vi "NRCToString.vi"(3 "SIDRQ":u8) -> (1 "NRC Message":string)   [LabVIEW 2011, in "Konvolucio MUDS150628.lvlib"]
uses:
  <instrlib>/Konvolucio MUDS150628/Konvolucio MUDS150628.lvlib
panel:
  out "NRC Num":T1(ring)=enum."noResponseFromSubnetComponent"
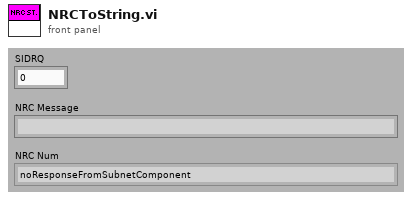
[diagram p1: front panel]
types:
  T1 = enum16{"generalReject", "serviceNotSupported", "subFunctionNotSupported", "incorrectMessageLengthOrInvalidFormat", "responseTooLong", "busyRepeatRequest", "conditionsNotCorrect", "requestSequenceError", "noResponseFromSubnetComponent", "failurePreventsExecutionOfRequestedAction", "requestOutOfRange", "securityAccessDenied", "invalidKey", "exceedNumberOfAttempts", "requiredTimeDelayNotExpired", "uploadDownloadNotAccepted", "transferDataSuspended", "generalProgrammingFailure", "wrongBlockSequenceCounter", "requestCorrectlyReceived", "subFunctionNotSupportedInActiveSession", "serviceNotSupportedInActiveSession", "rpmTooHigh", "rpmTooLow", "engineIsRunning", "engineIsNotRunning", "engineRunTimeTooLow", "temperatureTooHigh", "temperatureTooLow", "vehicleSpeedTooHigh", "vehicleSpeedTooLow", "throttle/PedalTooHigh", "throttle/PedalTooLow", "transmissionRangeNotInNeutral", "transmissionRangeNotInGear", "brakeSwitch(es)NotClosed", "shifterLeverNotInPark", "torqueConverterClutchLocked", "voltageTooHigh", "voltageTooLow", "undefined"}
  T2 = enum16{"generalReject", "serviceNotSupported", "subFunctionNotSupported", "incorrectMessageLengthOrInvalidFormat", "responseTooLong", "busyRepeatRequest", "conditionsNotCorrect", "requestSequenceError", "noResponseFromSubnetComponent", "failurePreventsExecutionOfRequestedAction", "requestOutOfRange", "securityAccessDenied", "invalidKey", "exceedNumberOfAttempts", "requiredTimeDelayNotExpired", "uploadDownloadNotAccepted", "transferDataSuspended", "generalProgrammingFailure", "wrongBlockSequenceCounter", "requestCorrectlyReceived", "subFunctionNotSupportedInActiveSession", "serviceNotSupportedInActiveSession", "rpmTooHigh", "rpmTooLow", "engineIsRunning", "engineIsNotRunning", "engineRunTimeTooLow", "temperatureTooHigh", "temperatureTooLow", "vehicleSpeedTooHigh", "vehicleSpeedTooLow", "throttle/PedalTooHigh", "throttle/PedalTooLow", "transmissionRangeNotInNeutral", "transmissionRangeNotInGear", "brakeSwitch(es)NotClosed", "shifterLeverNotInPark", "torqueConverterClutchLocked", "voltageTooHigh", "voltageTooLow"}
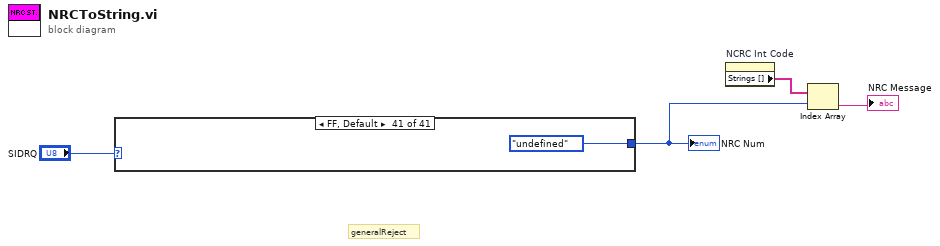
[diagram p0: block diagram]
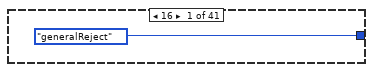
[diagram p2: hidden frame]
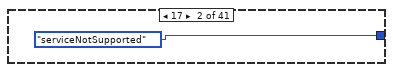
[diagram p3: hidden frame]
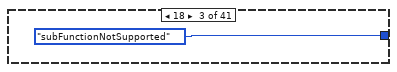
[diagram p4: hidden frame]
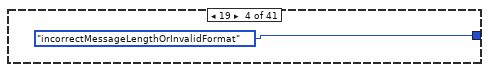
[diagram p5: hidden frame]
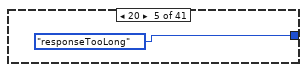
[diagram p6: hidden frame]
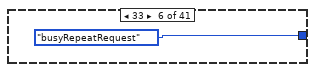
[diagram p7: hidden frame]
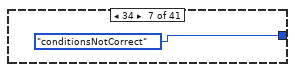
[diagram p8: hidden frame]
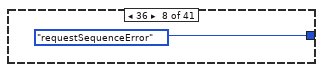
[diagram p9: hidden frame]
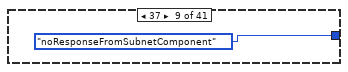
[diagram p10: hidden frame]
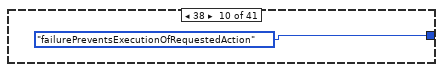
[diagram p11: hidden frame]
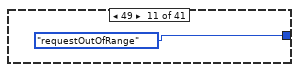
[diagram p12: hidden frame]
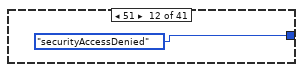
[diagram p13: hidden frame]
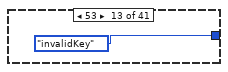
[diagram p14: hidden frame]
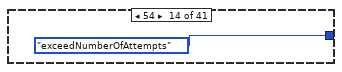
[diagram p15: hidden frame]
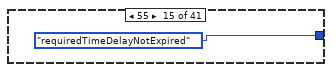
[diagram p16: hidden frame]
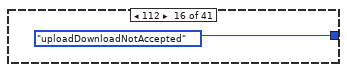
[diagram p17: hidden frame]
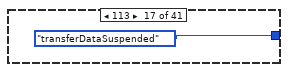
[diagram p18: hidden frame]
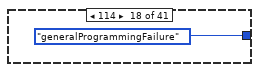
[diagram p19: hidden frame]
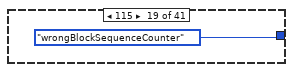
[diagram p20: hidden frame]
diagram:
  # "generalReject"
  n1 = case shown="FF, Default" "SIDRQ" {
    tunnel: [T2."generalReject" ("Enum") T2."serviceNotSupported" ("Enum") T2."subFunctionNotSupported" ("Enum") T2."incorrectMessageLengthOrInvalidFormat" ("Enum") T2."responseTooLong" ("Enum") T2."busyRepeatRequest" ("Enum") T2."conditionsNotCorrect" ("Enum") T2."requestSequenceError" ("Enum") T2."noResponseFromSubnetComponent" ("Enum") T2."failurePreventsExecutionOfRequestedAction" ("Enum") T2."requestOutOfRange" ("Enum") T2."securityAccessDenied" ("Enum") T2."invalidKey" ("Enum") T2."exceedNumberOfAttempts" ("Enum") T2."requiredTimeDelayNotExpired" ("Enum") T2."uploadDownloadNotAccepted" ("Enum") T2."transferDataSuspended" ("Enum") T2."generalProgrammingFailure" ("Enum") T2."wrongBlockSequenceCounter" ("Enum") T2."requestCorrectlyReceived" ("Enum") T2."subFunctionNotSupportedInActiveSession" ("Enum") T2."serviceNotSupportedInActiveSession" ("Enum") T2."rpmTooHigh" ("Enum") T2."rpmTooLow" ("Enum") T2."engineIsRunning" ("Enum") T2."engineIsNotRunning" ("Enum") T2."engineRunTimeTooLow" ("Enum") T2."temperatureTooHigh" ("Enum") T2."temperatureTooLow" ("Enum") T2."vehicleSpeedTooHigh" ("Enum") T2."vehicleSpeedTooLow" ("Enum") T2."throttle/PedalTooHigh" ("Enum") T2."throttle/PedalTooLow" ("Enum") T2."transmissionRangeNotInNeutral" ("Enum") T2."transmissionRangeNotInGear" ("Enum") T2."brakeSwitch(es)NotClosed" ("Enum") T2."shifterLeverNotInPark" ("Enum") T2."torqueConverterClutchLocked" ("Enum") T2."voltageTooHigh" ("Enum") T2."voltageTooHigh" ("Enum") T1."undefined" ("Enum")] -> w2
    frame 16 {
    }
    frame 17 {
    }
    frame 18 {
    }
    frame 19 {
    }
    frame 20 {
    }
    frame 33 {
    }
    frame 34 {
    }
    frame 36 {
    }
    frame 37 {
    }
    frame 38 {
    }
    frame 49 {
    }
    frame 51 {
    }
    frame 53 {
    }
    frame 54 {
    }
    frame 55 {
    }
    frame 112 {
    }
    frame 113 {
    }
    frame 114 {
    }
    frame 115 {
    }
    frame 120 {
    }
    frame 126 {
    }
    frame 127 {
    }
    frame 129 {
    }
    frame 130 {
    }
    frame 131 {
    }
    frame 132 {
    }
    frame 133 {
    }
    frame 134 {
    }
    frame 135 {
    }
    frame 136 {
    }
    frame 137 {
    }
    frame 138 {
    }
    frame 139 {
    }
    frame 140 {
    }
    frame 141 {
    }
    frame 143 {
    }
    frame 144 {
    }
    frame 145 {
    }
    frame 146 {
    }
    frame 147 {
    }
    frame 255, Default {
    }
  }
  "NRC Num" <- w2
  n2 = property on="NCRC Int Code" class="Enum (strict)"() -> ("Strings []"=w1:string[])  [unwired: 2 in, 2 out]
  n3 = Index Array(array=w1, index=w2) -> (element=→"NRC Message":string)
